vi "HCC Cycle Count Timer Update.vi"(6 "Timer Limit":dbl, 8 "Error In":errorcluster, 9 "Elapsed Time (sec)":dbl, 10 "Total Cycle Count (Current) OUT":u16, 11 "Input Cycle Count OUT in":u16) -> (0 "Error Out":errorcluster, 3 "Input Cycle Count OUT out":u16)   [LabVIEW 2016]
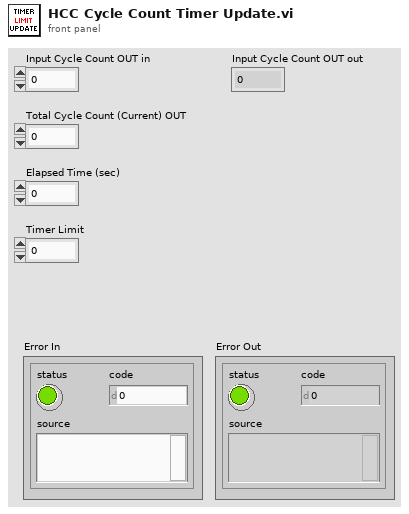
[diagram p1: front panel]
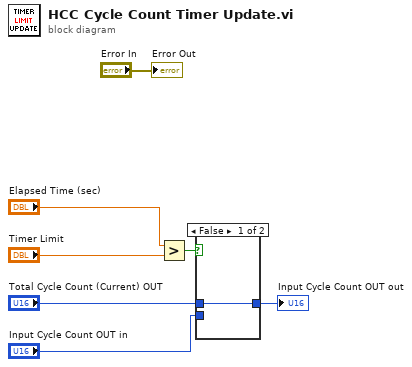
[diagram p0: block diagram]
diagram:
  n1 = Greater?(x="Elapsed Time (sec)", y="Timer Limit") -> (0:w5:bool)
  n2 = case shown="False" w5 {
    tunnel: "Total Cycle Count (Current) OUT" -> [w8 _]
    tunnel: [w8 w9] -> w4
    tunnel: "Input Cycle Count OUT in" -> [_ w9]
    frame False {
    }
    frame True {
    }
  }
  "Input Cycle Count OUT out" <- w4
  "Error Out" <- "Error In"
